vi "Initialize.vi"(8 "error in (no error)":errorcluster, 11 "NHRDCPower in":refnum<class "NHRDCPower.lvclass">) -> (0 "error out":errorcluster, 3 "NHRDCPower out":refnum<class "NHRDCPower.lvclass">)   [LabVIEW 2018, in "AcPwrPlugins.lvlib" / "NHRDCPower.lvclass"]
doc: "This VI establishes communication to the instrument and may provide other functions such as reset the instrument or provide a range check."
uses:
  NHRDCPower.lvclass
  <instrlib>/NHRDCPowerModule/NHRDCPowerModule/NHRDCPowerModule.lvlib
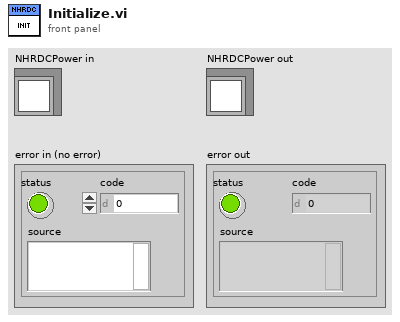
[diagram p1: front panel]
types:
  T1 = cluster{"f":bool, "instrument handle out":refnum<visa-resource-name>}[]
  T2 = typedef "AcPwrPlugins.lvlib/NHRDCPower.lvclass/Device(s)Settings.ctl" = cluster{"Handle":string, "Name":string, "Phase Select":i32, "id query (Yes)":bool, "reset device (Yes)":bool, "Connected":bool, "Voltage Range (V)":dbl[], "Timing":cluster{"TimingOn":enum16{""}, "Hours":u32, "Minutes":u32, "Seconds":dbl, "CutoffVoltage":dbl}, "Simulate Instrument(T)":bool, "SlewRate":cluster{"Set Voltage Rate V/S":dbl, "Set Current Rate A/S":dbl, "Set Resistance Rate R/S":dbl, "Set Power Rate W/S":dbl}, "OutputSettings":cluster{"operating state (Off)":i32, "Voltage (V)":dbl, "Current (A)":dbl, "Resistance (Ohms)":dbl, "Power (W)":dbl, "Enable Voltage":bool, "Enable Current":bool, "Enable Resistance":bool, "Enable Power":bool}}[]
  T3 = cluster{"f":bool, "instrument handle out":refnum<visa-resource-name>}
  T4 = cluster{"Handle":string, "Name":string, "Phase Select":i32, "id query (Yes)":bool, "reset device (Yes)":bool, "Connected":bool, "Voltage Range (V)":dbl[], "Timing":cluster{"TimingOn":enum16{""}, "Hours":u32, "Minutes":u32, "Seconds":dbl, "CutoffVoltage":dbl}, "Simulate Instrument(T)":bool, "SlewRate":cluster{"Set Voltage Rate V/S":dbl, "Set Current Rate A/S":dbl, "Set Resistance Rate R/S":dbl, "Set Power Rate W/S":dbl}, "OutputSettings":cluster{"operating state (Off)":i32, "Voltage (V)":dbl, "Current (A)":dbl, "Resistance (Ohms)":dbl, "Power (W)":dbl, "Enable Voltage":bool, "Enable Current":bool, "Enable Resistance":bool, "Enable Power":bool}}
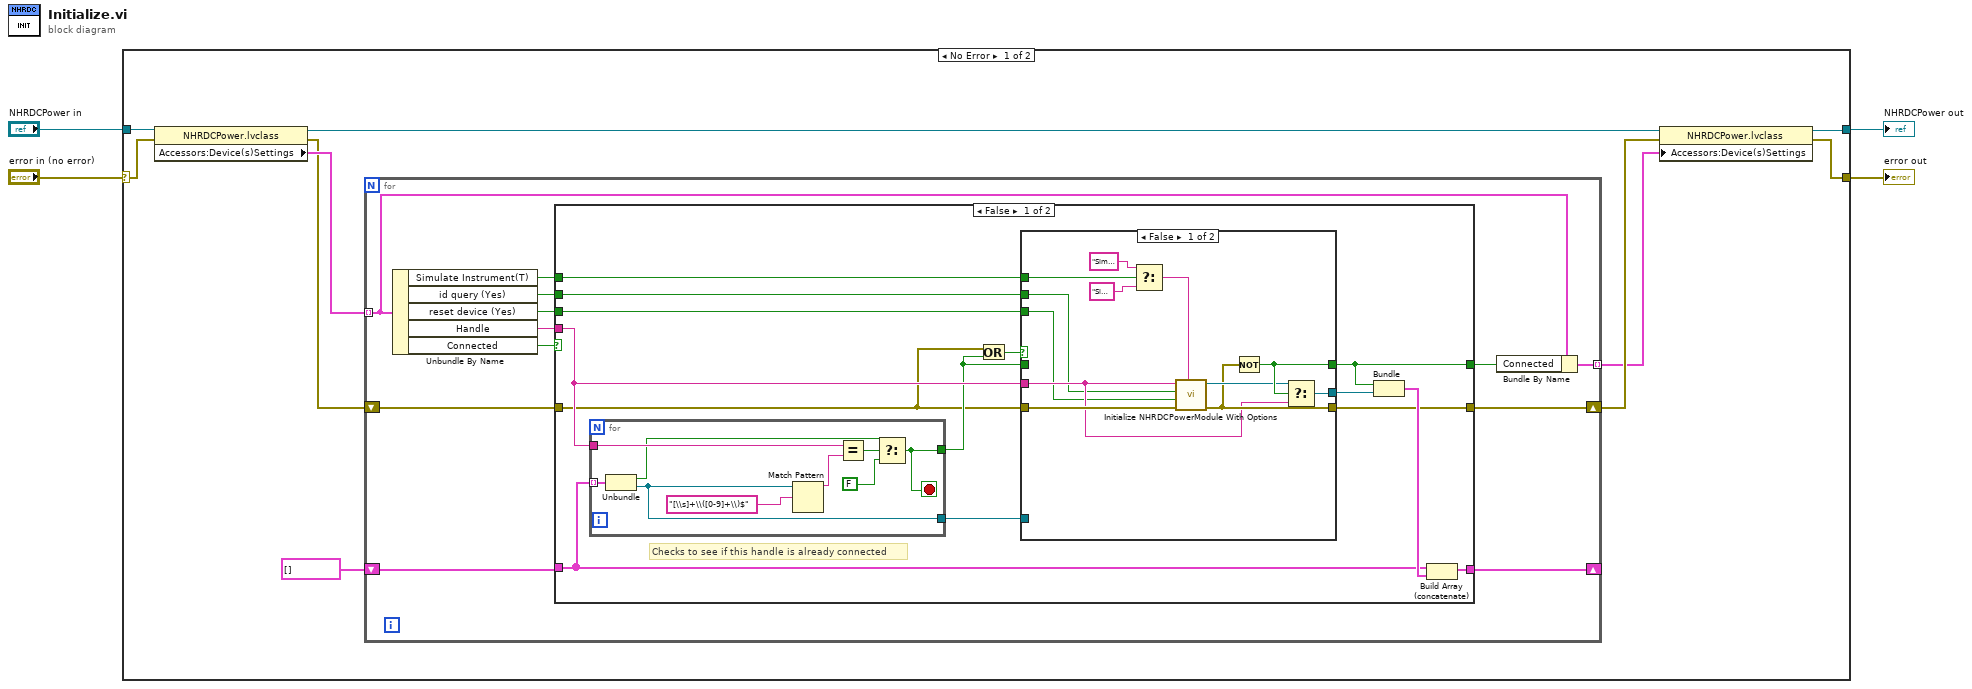
[diagram p0: block diagram]
diagram:
  n1 = case shown="No Error" "error in (no error)" {
    selector: "error in (no error)" -> [w13 w68]
    tunnel: "NHRDCPower in" -> [w14 w69]
    tunnel: [w9 w69] -> w2
    tunnel: [w6 w68] -> w1
    frame No Error {
      n2 = property class="NHRDCPower.lvclass"(reference=w14, error in=w13) -> (reference out=w12:refnum<class "NHRDCPower.lvclass">, error out=w10:errorcluster, "Accessors:Device(s)Settings"=w11:T2)
      n3 = for {
        shift-right: [w25] -> w8
        shift-left: w10 -> [w26]
        tunnel: w11 -> [w19] mode=indexing
        shift-right: [w23] -> _
        shift-left: T1 [] -> [w24]
        tunnel: [w18] -> w7 mode=indexing
        n4 = Unbundle By Name(w19) -> ("Simulate Instrument(T)"=w17:bool, "id query (Yes)"=w16:bool, "reset device (Yes)"=w15:bool, "Handle"=w22:string, "Connected"=w21:bool)
        n5 = case shown="False" w21 {
          selector: w21 -> [_ w67]
          tunnel: [w31 w67] -> w20
          tunnel: w22 -> [w40 _]
          tunnel: [w32 w66] -> w25
          tunnel: w26 -> [w30 w66]
          tunnel: w24 -> [w33 w65]
          tunnel: [w37 w65] -> w23
          tunnel: w17 -> [w29 _]
          tunnel: w16 -> [w28 _]
          tunnel: w15 -> [w27 _]
          frame False {
            # "Checks to see if this handle is already connected"
            n6 = for {
              tunnel: w40 -> [w49]
              tunnel: [w47] -> w38
              tunnel: w33 -> [w43] mode=indexing
              tunnel: [w41] -> w34
              stop <- w47 stop-if-true
              n7 = Unbundle(w43) -> ("f"=w42:bool, "instrument handle out"=w41:refnum<visa-resource-name>)
              n8 = Match Pattern(string=w41, regular expression="[\\s]+\\([0-9]+\\)$") -> (before substring=w45:string)  [unwired: 1 in, 3 out]
              n9 = Equal?(x=w49, y=w45) -> (x = y?=w48:bool)
              n10 = Select(t=w42, s=w48, f=FALSE) -> (s? t:f=w47:bool)
            }
            n11 = Or(x=w30, y=w38) -> (x .or. y?=w39:bool)
            n12 = case shown="False" w39 {
              tunnel: [w60 w63] -> w31
              tunnel: w40 -> [w56 _]
              tunnel: w30 -> [w57 w64]
              tunnel: [w58 w64] -> w32
              tunnel: w38 -> [_ w63]
              tunnel: [w61 w62] -> w36
              tunnel: w34 -> [_ w62]
              tunnel: w29 -> [w51 _]
              tunnel: w28 -> [w55 _]
              tunnel: w27 -> [w54 _]
              frame False {
                n13 = Select(t="Simulate=1,RangeCheck=1,QueryInstrStatus=1,Cache=0" ("Option String"), s=w51, f="Simulate=0,RangeCheck=1,QueryInstrStatus=1,Cache=0" ("Option String")) -> (s? t:f=w50:string)
                n14 = call <instrlib>:"Initialize NHRDCPowerModule With Options.vi"("options"=w50, "error in (no error)"=w57, "reset device (Off)"=w54, "id query (Off)"=w55, "resource name"=w56) -> ("error out"=w58:errorcluster, "instrument handle out"=w59:refnum<visa-resource-name>)  [unwired: 5 in]
                n15 = Not(x=w58) -> (.not. x?=w60:bool)
                n16 = Select(t=w59, s=w60, f=w56) -> (s? t:f=w61:refnum<visa-resource-name>)
              }
              frame True {
              }
            }
            n17 = Bundle("f"=w31, "instrument handle out"=w36) -> (w35:T3)  [unwired: 1 in]
            n18 = Build Array (concatenate)(w33, w35) -> (w37:T1)
          }
          frame True {
          }
        }
        n19 = Bundle By Name(cluster=w19, "Connected"=w20) -> (w18:T4)
      }
      n20 = property class="NHRDCPower.lvclass"(reference=w12, error in=w8, "Accessors:Device(s)Settings"=w7) -> (reference out=w9:refnum<class "NHRDCPower.lvclass">, error out=w6:errorcluster)
    }
    frame Error {
    }
  }
  "error out" <- w1
  "NHRDCPower out" <- w2
